vi "GetStimMode.vi"(0 "VISA Resource Name":refnum<visa-resource-name>="COM1", 5 "DeviceInitializationEnable":bool, 11 "error in (no error)":errorcluster) -> (3 "Status":string, 4 "VISA resource name out":refnum<visa-resource-name>, 6 "Start Mode":bool=TRUE, 8 "Stimulation Initialized":bool=TRUE, 10 "Stimulation Started":bool=TRUE, 14 "error out":errorcluster, 15 "Transfer/Busy Error":bool=TRUE)   [LabVIEW 2020]
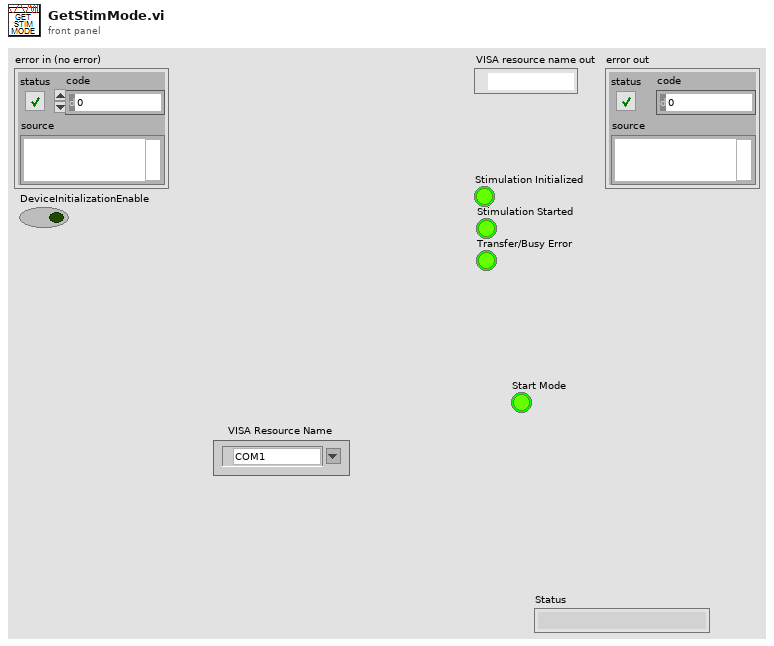
[diagram p1: front panel]
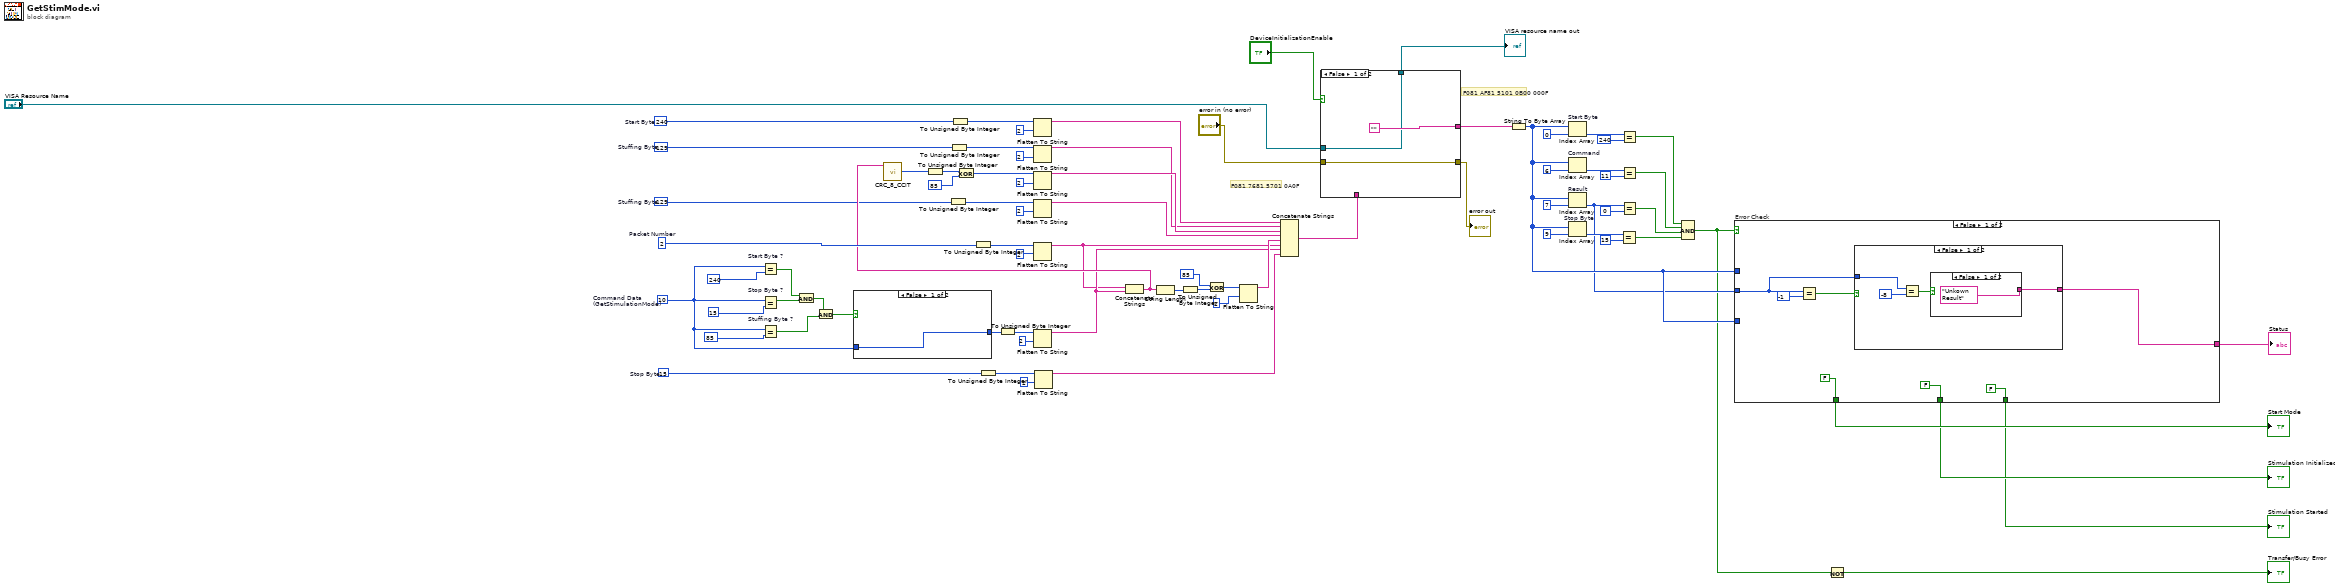
[diagram p0: block diagram]
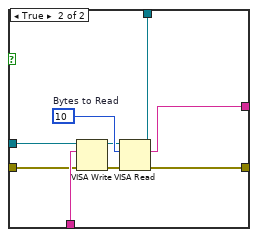
[diagram p2: hidden frame]
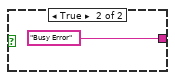
[diagram p3: hidden frame]
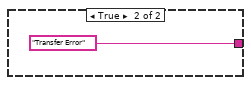
[diagram p4: hidden frame]
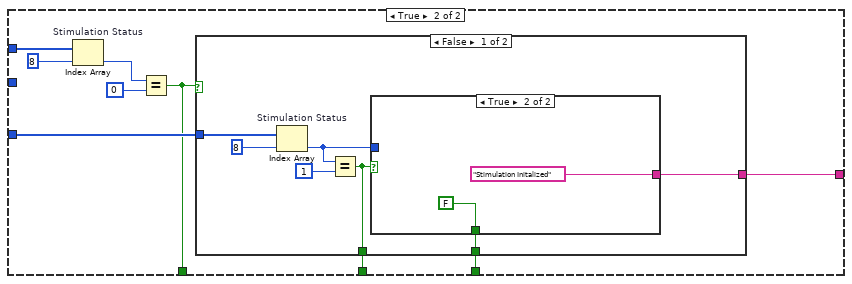
[diagram p5: hidden frame]
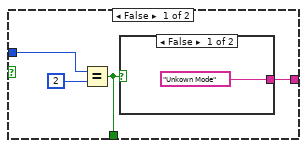
[diagram p6: hidden frame]
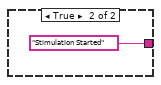
[diagram p7: hidden frame]
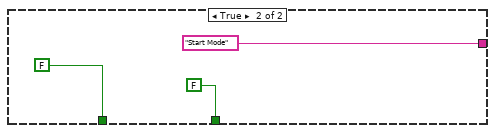
[diagram p8: hidden frame]
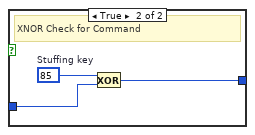
[diagram p9: hidden frame]
diagram:
  w75 = u8 2  # Packet Number
  w40 = 15  # Stop Byte
  w43 = 129  # Stuffing Byte
  w44 = 129  # Stuffing Byte
  w42 = 240  # Start Byte
  w58 = 10  # Command Data (GetStimulationMode)
  # "F081 7681 5701 0A0F"
  # "F081 AF81 5101 0B00 000F"
  n1 = Equal? "Start Byte ?"(x=w58, y=240 ("IntAck")) -> (x = y?=w31:bool)
  n2 = Equal? "Stop Byte ?"(x=w58, y=15 ("IntAck")) -> (x = y?=w32:bool)
  n3 = Equal? "Stuffing Byte ?"(x=w58, y=85 ("IntAck")) -> (x = y?=w34:bool)
  n4 = And(x=w31, y=w32) -> (x .and. y?=w33:bool)
  n5 = And(x=w33, y=w34) -> (x .and. y?=w35:bool)
  n6 = case shown="False" w35 {
    tunnel: w58 -> [w77 w80]
    tunnel: [w77 w78] -> w59
    frame False {
    }
    frame True {
      w79 = 85  # Stuffing key
      # "XNOR Check for Command"
      n7 = Exclusive Or(1:w80, 2:w79) -> (0:w78:i32)
    }
  }
  n8 = To Unsigned Byte Integer(number=w44) -> (unsigned 8bit integer=w47:u8)
  n9 = To Unsigned Byte Integer(number=w43) -> (unsigned 8bit integer=w46:u8)
  n10 = To Unsigned Byte Integer(number=w42) -> (unsigned 8bit integer=w45:u8)
  n11 = To Unsigned Byte Integer(number=w75) -> (unsigned 8bit integer=w66:u8)
  n12 = To Unsigned Byte Integer(number=w40) -> (unsigned 8bit integer=w41:u8)
  n13 = To Unsigned Byte Integer(number=w59) -> (unsigned 8bit integer=w65:u8)
  n14 = Flatten To String(anything=w45, byte order (0:big-endian, network order)=2) -> (data string=w36:string)  [unwired: 2 in, 2 out]
  n15 = Flatten To String(anything=w46, byte order (0:big-endian, network order)=2) -> (data string=w37:string)  [unwired: 2 in, 2 out]
  n16 = Flatten To String(anything=w47, byte order (0:big-endian, network order)=2) -> (data string=w39:string)  [unwired: 2 in, 2 out]
  n17 = Flatten To String(anything=w66, byte order (0:big-endian, network order)=2) -> (data string=w60:string)  [unwired: 2 in, 2 out]
  n18 = Flatten To String(anything=w65, byte order (0:big-endian, network order)=2) -> (data string=w61:string)  [unwired: 2 in, 2 out]
  n19 = Flatten To String(anything=w41, byte order (0:big-endian, network order)=2) -> (data string=w30:string)  [unwired: 2 in, 2 out]
  n20 = Concatenate Strings(w60, w61) -> (w68:string)
  n21 = call "CRC_8_CCIT.vi"("Data String"=w68) -> ("Numeric"=w67:u8)  [unwired: 10 in]
  n22 = To Unsigned Byte Integer(number=w67) -> (unsigned 8bit integer=w70:u8)
  n23 = Exclusive Or(1:u8 85, 2:w70) -> (0:w69:u8)
  n24 = Flatten To String(anything=w69, byte order (0:big-endian, network order)=2) -> (data string=w38:string)  [unwired: 2 in, 2 out]
  n25 = String Length(string=w68) -> (length=w63:i32)
  n26 = To Unsigned Byte Integer(number=w63) -> (unsigned 8bit integer=w73:u8)
  n27 = Exclusive Or(1:w73, 2:u8 85) -> (0:w72:u8)
  n28 = Flatten To String(anything=w72, byte order (0:big-endian, network order)=2) -> (data string=w64:string)  [unwired: 2 in, 2 out]
  n29 = Concatenate Strings(w36, w37, w38, w39, w64, w60, w61, w30) -> (w6:string)
  n30 = case shown="False" "DeviceInitializationEnable" {
    tunnel: "VISA Resource Name" -> [w82 w89]
    tunnel: w6 -> [_ w88]
    tunnel: ["" w87] -> w5
    tunnel: "error in (no error)" -> [w81 w86]
    tunnel: [w81 w85] -> w2
    tunnel: [w82 w84] -> w1
    frame False {
    }
    frame True {
      w92 = 10  # Bytes to Read
      n31 = VISA Write(VISA resource name=w89, write buffer=w88, error in (no error)=w86) -> (VISA resource name out=w91:refnum<visa-resource-name>, error out=w90:errorcluster)  [unwired: 1 out]
      n32 = VISA Read(VISA resource name=w91, byte count=w92, error in (no error)=w90) -> (VISA resource name out=w84:refnum<visa-resource-name>, read buffer=w87:string, error out=w85:errorcluster)  [unwired: 1 out]
    }
  }
  "VISA resource name out" <- w1
  "error out" <- w2
  n33 = String To Byte Array(string=w5) -> (unsigned byte array=w14:u8[])
  n34 = Index Array "Start Byte"(array=w14, index=0) -> (element=w25:u8)
  n35 = Index Array "Command"(array=w14, index=6) -> (element=w23:u8)
  n36 = Index Array "Result"(array=w14, index=7) -> (element=w13:u8)
  n37 = Index Array "Stop Byte"(array=w14, index=9) -> (element=w20:u8)
  n38 = Equal?(x=w20, y=u16 15) -> (x = y?=w15:bool)
  n39 = Equal?(x=w25, y=u16 240) -> (x = y?=w16:bool)
  n40 = Equal?(x=w23, y=u16 11) -> (x = y?=w17:bool)
  n41 = Equal?(x=w13, y=u16 0) -> (x = y?=w18:bool)
  n42 = Compound Arithmetic op=AND(w16, w17, w18, w15) -> (w9:bool)
  n43 = case "Error Check" shown="False" w9 {
    tunnel: w14 -> [_ w114]
    tunnel: [w97 w111] -> w76
    tunnel: w14 -> [_ w110]
    tunnel: w13 -> [w96 _]
    tunnel: [FALSE w109] -> w12
    tunnel: [FALSE w108] -> w11
    tunnel: [FALSE w107] -> w10
    frame False {
      n44 = Equal?(x=w96, y=i8 -1) -> (x = y?=w98:bool)
      n45 = case shown="False" w98 {
        tunnel: [w103 "Transfer Error"] -> w97
        tunnel: w96 -> [w101 _]
        frame False {
          n46 = Equal?(x=w101, y=i8 -8) -> (x = y?=w100:bool)
          n47 = case shown="False" w100 {
            tunnel: ["Unkown Result" "Busy Error"] -> w103
            frame False {
            }
            frame True {
            }
          }
        }
        frame True {
        }
      }
    }
    frame True {
      n48 = Index Array "Stimulation Status"(array=w114, index=8) -> (element=w112:u8)
      n49 = Equal?(x=w112, y=u16 0) -> (x = y?=w109:bool)
      n50 = case shown="False" w109 {
        tunnel: [w119 "Start Mode"] -> w111
        tunnel: w110 -> [w122 _]
        tunnel: [w117 FALSE] -> w108
        tunnel: [w116 FALSE] -> w107
        frame False {
          n51 = Index Array "Stimulation Status"(array=w122, index=8) -> (element=w118:u8)
          n52 = Equal?(x=w118, y=u16 1) -> (x = y?=w117:bool)
          n53 = case shown="True" w117 {
            tunnel: [w126 "Stimulation Initalized"] -> w119
            tunnel: w118 -> [w124 _]
            tunnel: [w123 FALSE] -> w116
            frame False {
              n54 = Equal?(x=w124, y=u16 2) -> (x = y?=w123:bool)
              n55 = case shown="False" w123 {
                tunnel: ["Unkown Mode" "Stimulation Started"] -> w126
                frame False {
                }
                frame True {
                }
              }
            }
            frame True {
            }
          }
        }
        frame True {
        }
      }
    }
  }
  "Status" <- w76
  "Start Mode" <- w12
  "Stimulation Initialized" <- w11
  "Stimulation Started" <- w10
  n56 = Not(x=w9) -> (.not. x?=→"Transfer/Busy Error":bool)
